vi "Handle EVENT.vi"(8 "error in (no error)":errorcluster, 9 "Message Loop Data (in)":T1, 10 "Cluster":T14 {"Message Codes" items=["HELLO"=1, "WELCOME"=2, "ABORT"=3, "GOODBYE"=6, "ERROR"=8, "PUBLISH"=16, "PUBLISHED"=17, "SUBSCRIBE"=32, "SUBSCRIBED"=33, "UNSUBSCRIBE"=34, "UNSUBSCRIBED"=35, "EVENT"=36, "CALL"=48, "RESULT"=59, "REGISTER"=64, "REGISTERED"=65, "UNREGISTER"=66, "UNREGISTERED"=67, "INVOCATION"=68, "YIELD"=70]}, 11 "reference":refnum<class "WAMP Client.lvclass">) -> (0 "error out":errorcluster, 1 "Message Loop Data (out)":T1, 3 "reference out":refnum<class "WAMP Client.lvclass">)   [LabVIEW 2020, in "wamplv.lvlib" / "WAMP Client.lvclass"]
uses:
  <vilib>/samangh/wamplv/WAMP Client/WAMP Client.lvclass
  <vilib>/samangh/wamplv/WAMP Client/TypeDef/WAMP Received Message.ctl
  <vilib>/samangh/wamplv/WAMP Message Codes.ctl
  <vilib>/samangh/wamplv/WAMP Client/TypeDef/Message Loop Shift Reg Data.ctl
  <vilib>/samangh/wamplv/WAMP Client/TypeDef/REGISTER Request Data.ctl
  <vilib>/samangh/wamplv/WAMP Client/TypeDef/REGISTERED or ERROR payload.ctl
  <vilib>/samangh/wamplv/WAMP Client/TypeDef/Combined error.ctl
  <vilib>/samangh/wamplv/WAMP Client/TypeDef/WAMP Error Payload.ctl
  <vilib>/samangh/wamplv/WAMP Client/TypeDef/INVOCATION payload.ctl
  <vilib>/samangh/wamplv/WAMP Client/TypeDef/Publish Requests Map.ctl
  <vilib>/samangh/wamplv/WAMP Client/TypeDef/PUBLISH Request Data.ctl
  <vilib>/samangh/wamplv/WAMP Client/TypeDef/PUBLISH Result.ctl
  <vilib>/samangh/wamplv/WAMP Client/TypeDef/Endpoint Data.ctl
  <vilib>/samangh/wamplv/WAMP Client/TypeDef/CALL Request Map.ctl
  <vilib>/samangh/wamplv/WAMP Client/TypeDef/CALL Request Data.ctl
  <vilib>/samangh/wamplv/WAMP Client/TypeDef/RESULT Payload.ctl
  <vilib>/samangh/wamplv/WAMP Client/TypeDef/SUBSCRIBE Requests Map.ctl
  <vilib>/samangh/wamplv/WAMP Client/TypeDef/SUBSCRIBE Request Data.ctl
  <vilib>/samangh/wamplv/WAMP Client/TypeDef/Subscribe Result.ctl
  <vilib>/samangh/wamplv/WAMP Client/TypeDef/Event Payload.ctl
  <vilib>/samangh/wamplv/WAMP Client/TypeDef/Subscriptions Map.ctl
  <vilib>/samangh/wamplv/WAMP Client/TypeDef/Subscription Details.ctl
  <vilib>/samangh/wamplv/WAMP Client/TypeDef/Unsubscribe Requests Map.ctl
  <vilib>/samangh/wamplv/WAMP Client/TypeDef/UNSUBSCRIBE Request Data.ctl
  <vilib>/samangh/wamplv/WAMP Client/TypeDef/UNSUBSCRIBE Result.ctl
  <vilib>/samangh/wamplv/WAMP Client/WAMP Client.lvclass/WAMP Client.ctl
  <vilib>/JDP Science/JSONtext/JSONtext.lvlib
panel:
  out "Details":string
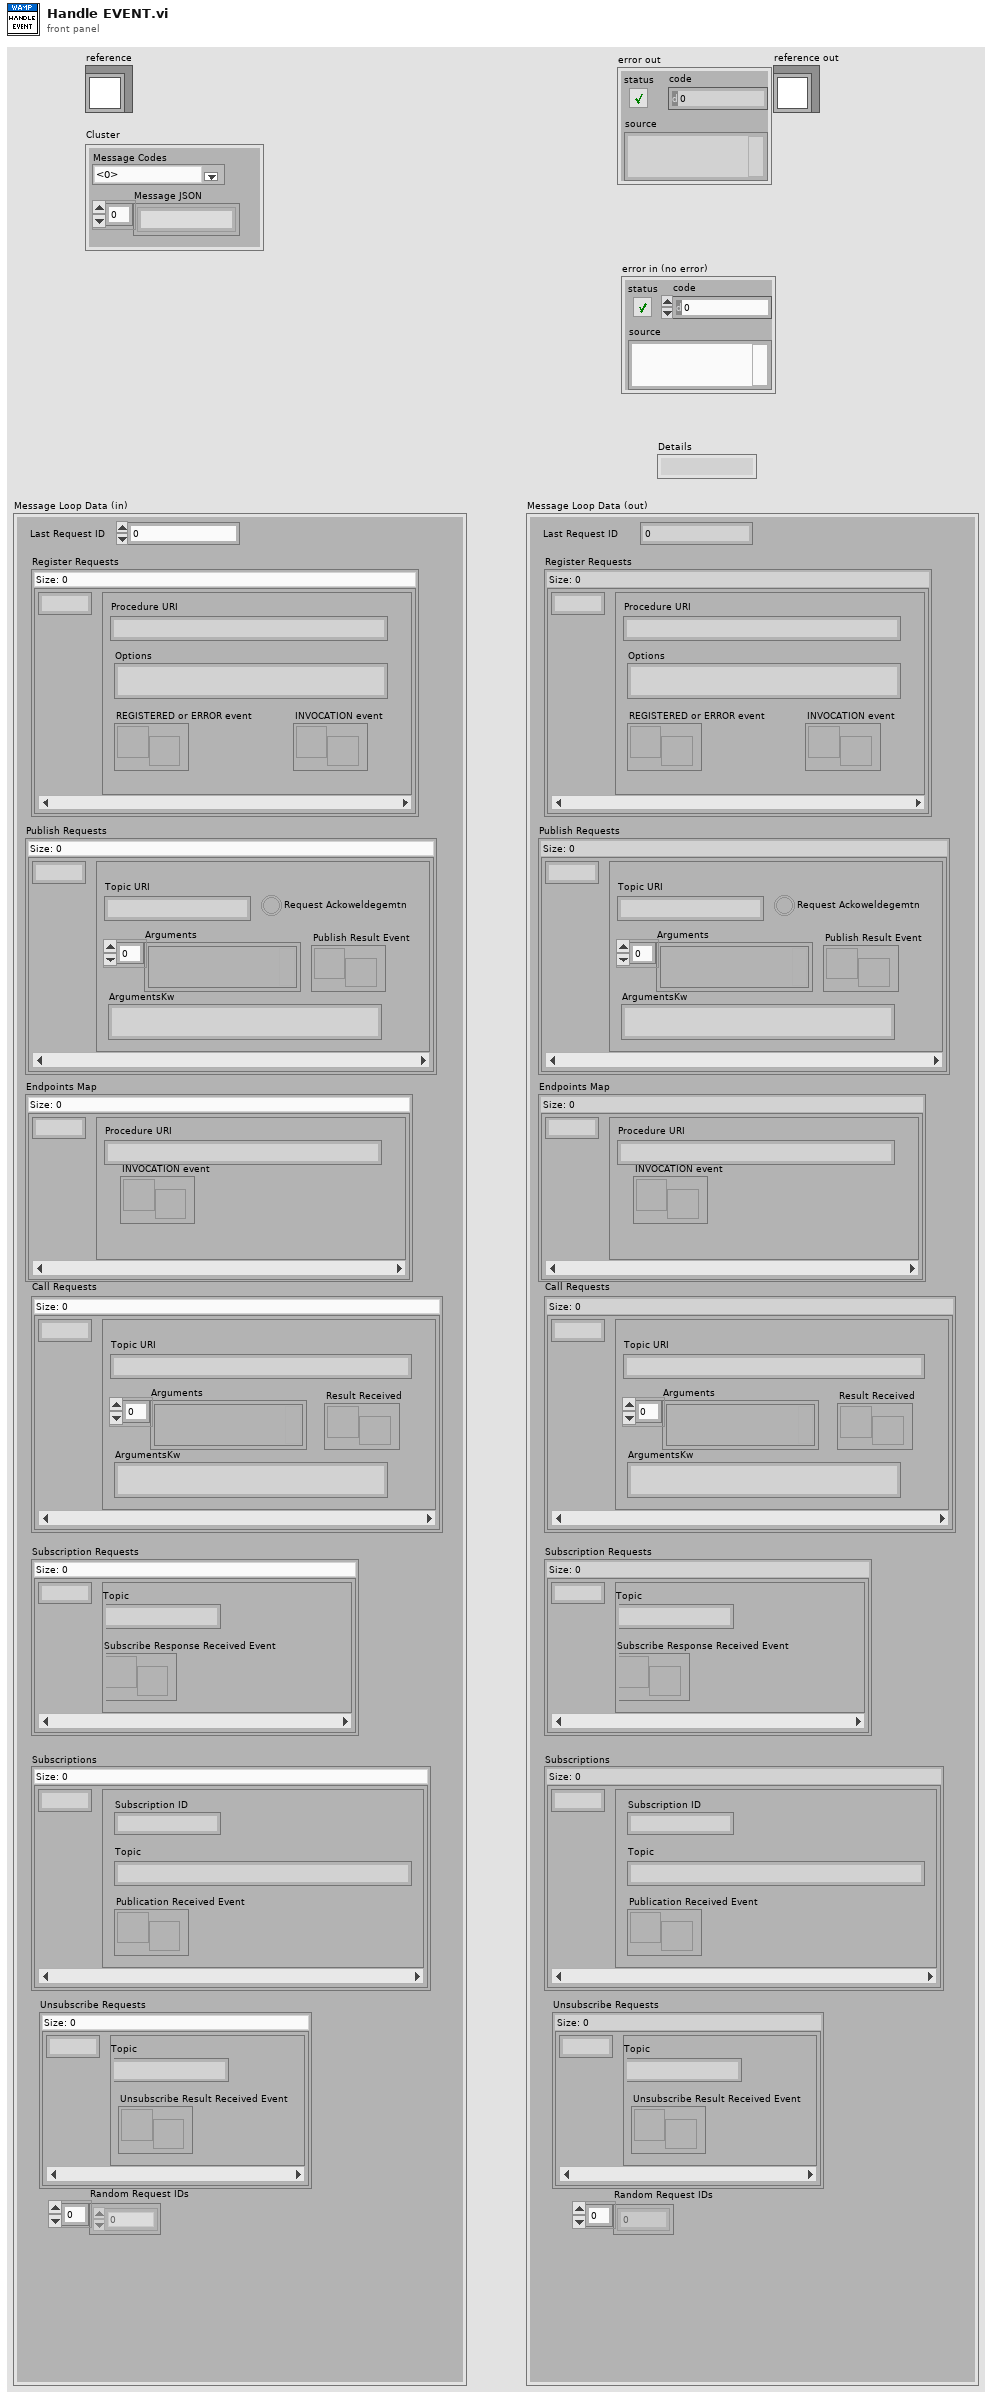
[diagram p1: front panel]
types:
  T1 = typedef "wamplv.lvlib/WAMP Client.lvclass/Message Loop Shift Reg Data.ctl" = cluster{"Last Request ID":u64, "Register Requests":map{u64, T2}, "Publish Requests":T3, "Endpoints Map":map{u64, T5}, "Call Requests":T6, "Subscription Requests":T8, "Subscriptions":T10, "Unsubscribe Requests":T12, "Random Request IDs":u64[]}
  T2 = typedef "wamplv.lvlib/WAMP Client.lvclass/REGISTER Request Data.ctl" = cluster{"Procedure URI":string, "Options":string, "REGISTERED or ERROR event":refnum<user-event>, "INVOCATION event":refnum<user-event>}
  T3 = typedef "wamplv.lvlib/WAMP Client.lvclass/Publish Requests Map.ctl" = map{u64, T4}
  T4 = typedef "wamplv.lvlib/WAMP Client.lvclass/PUBLISH Request Data.ctl" = cluster{"Topic URI":string, "Arguments":variant[], "ArgumentsKw":string, "Publish Result Event":refnum<user-event>, "Request Ackoweldegemtn":bool}
  T5 = typedef "wamplv.lvlib/WAMP Client.lvclass/Endpoint Data.ctl" = cluster{"Procedure URI":string, "INVOCATION event":refnum<user-event>}
  T6 = typedef "wamplv.lvlib/WAMP Client.lvclass/CALL Request Map.ctl" = map{u64, T7}
  T7 = typedef "wamplv.lvlib/WAMP Client.lvclass/CALL Request Data.ctl" = cluster{"Topic URI":string, "Arguments":variant[], "ArgumentsKw":string, "Result Received":refnum<user-event>}
  T8 = typedef "wamplv.lvlib/WAMP Client.lvclass/SUBSCRIBE Requests Map.ctl" = map{u64, T9}
  T9 = typedef "wamplv.lvlib/WAMP Client.lvclass/SUBSCRIBE Request Data.ctl" = cluster{"Topic":string, "Subscribe Response Received Event":refnum<user-event>}
  T10 = typedef "wamplv.lvlib/WAMP Client.lvclass/Subscriptions Map.ctl" = map{u64, T11}
  T11 = typedef "wamplv.lvlib/WAMP Client.lvclass/Subscription Details.ctl" = cluster{"Subscription ID":u64, "Topic":string, "Publication Received Event":refnum<user-event>}
  T12 = typedef "wamplv.lvlib/WAMP Client.lvclass/Unsubscribe Requests Map.ctl" = map{u64, T13}
  T13 = typedef "wamplv.lvlib/WAMP Client.lvclass/UNSUBSCRIBE Request Data.ctl" = cluster{"Topic":string, "Unsubscribe Result Received Event":refnum<user-event>}
  T14 = typedef "wamplv.lvlib/WAMP Client.lvclass/WAMP Received Message.ctl" = cluster{"Message JSON":string[], "Message Codes":T15}
  T15 = typedef "wamplv.lvlib/WAMP Client.lvclass/WAMP Message Codes.ctl" = u16
  T16 = typedef "wamplv.lvlib/WAMP Client.lvclass/Event Payload.ctl" = cluster{"Arguments Payload":string[], "ArgumentKw Payload":string, "Topic":string}
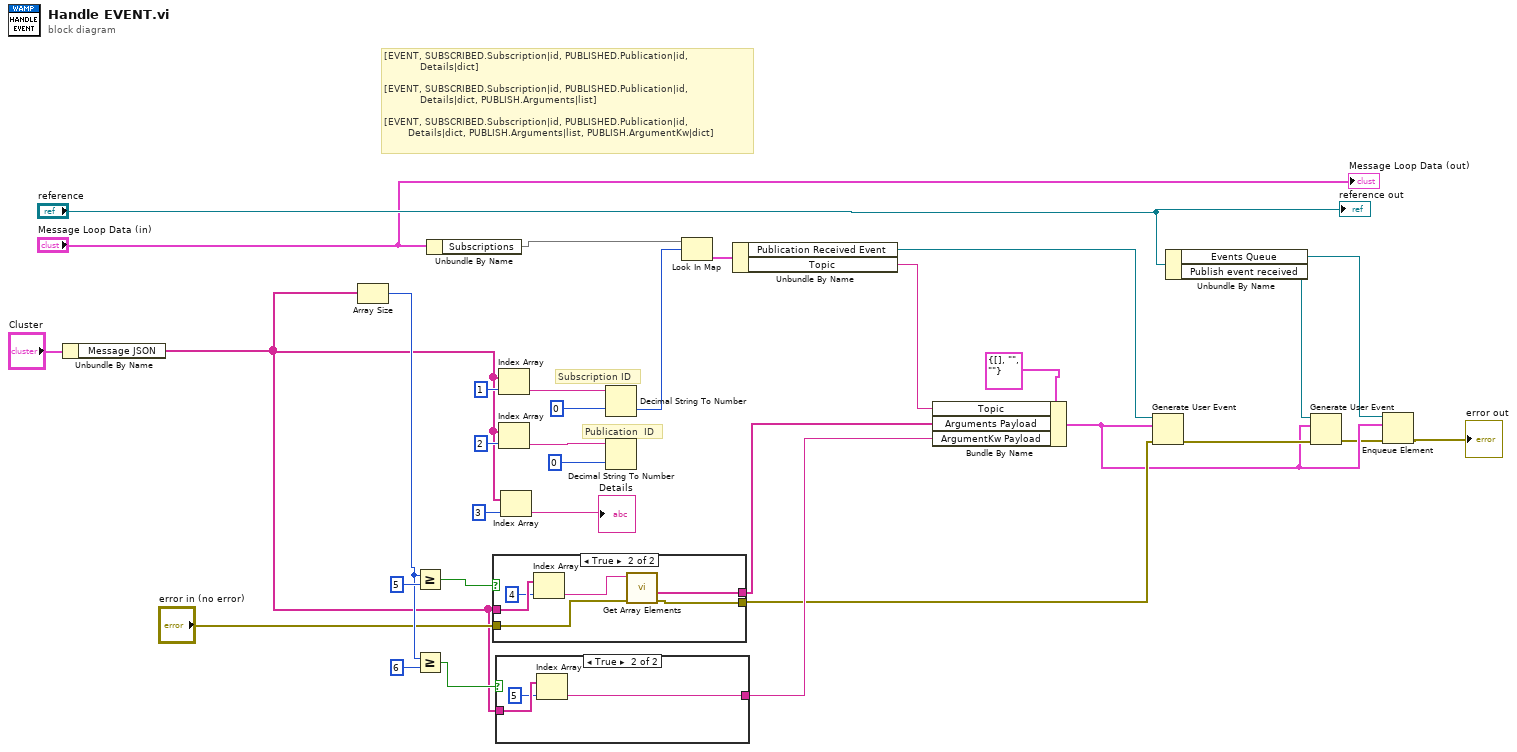
[diagram p0: block diagram]
diagram:
  # "[EVENT, SUBSCRIBED.Subscription|id, PUBLISHED.Publication|id,\n            Details|dict]\n\n[EVENT, SUBSCRIBED.Subscription|id, PUBLISHED.Publication|id,\n            Details|dict, PUBLISH.Arguments|list]\n\n[EVENT, SUBSCRIBED.Subscription|id, PUBLISHED.Publication|id,\n        Details|dict, PUBLISH.Arguments|list, PUBLISH.ArgumentKw|dict]"
  # "Publication  ID"
  # "Subscription ID"
  n1 = Unbundle By Name("Cluster") -> ("Message JSON"=w15:string[])
  n2 = Array Size(array=w15) -> (size(s)=w21:i32)
  n3 = Greater Or Equal?(x=w21, y=5) -> (x >= y?=w24:bool)
  n4 = Greater Or Equal?(x=w21, y=6) -> (x >= y?=w19:bool)
  n5 = Unbundle By Name("Message Loop Data (in)") -> ("Subscriptions"=w2:T10)
  n6 = case shown="True" w24 {
    tunnel: w15 -> [_ w39]
    tunnel: [_ w37] -> w23
    tunnel: "error in (no error)" -> [w34 w36]
    tunnel: [w34 w35] -> w17
    frame False {
    }
    frame True {
      n7 = Index Array(array=w39, index=4) -> (element=w40:string)
      n8 = call <vilib>:"Get Array Elements.vi"("error in (no error)"=w36, "JSON"=w40) -> ("error out"=w35:errorcluster, "<JSON>"=w37:string[])  [unwired: 7 in, 1 out]
    }
  }
  n9 = case shown="True" w19 {
    tunnel: w15 -> [_ w43]
    tunnel: [_ w41] -> w20
    frame False {
    }
    frame True {
      n10 = Index Array(array=w43, index=5) -> (element=w41:string)
    }
  }
  n11 = Index Array(array=w15, index=1) -> (element=w32:string)
  n12 = Index Array(array=w15, index=2) -> (element=w33:string)
  n13 = Index Array(array=w15, index=3) -> (element=→"Details":string)
  n14 = Decimal String To Number(string=w32, default (0L)=u64 0) -> (number=w14:u64)  [unwired: 1 in, 1 out]
  n15 = Decimal String To Number(string=w33, default (0L)=u64 0) -> ()  [unwired: 1 in, 2 out]
  n16 = Look In Map(map=w2, key=w14) -> (value=w13:T11)  [unwired: 1 in, 1 out]
  n17 = Unbundle By Name(w13) -> ("Publication Received Event"=w12:refnum<user-event>, "Topic"=w11:string)
  n18 = Bundle By Name(cluster=T16 {"Arguments Payload"=[], "ArgumentKw Payload"="", "Topic"=""} ("Cluster"), "Topic"=w11, "Arguments Payload"=w23, "ArgumentKw Payload"=w20) -> (w5:T16)
  n19 = Generate User Event(user event=w12, event data cluster=w5, error in=w17) -> (error out=w7:errorcluster)  [unwired: 1 in, 1 out]
  n20 = Unbundle By Name("reference") -> ("Events Queue"=w6:refnum<queue>, "Publish event received"=w9:refnum<user-event>)
  n21 = Generate User Event(user event=w9, event data cluster=w5, error in=w7) -> (error out=w4:errorcluster)  [unwired: 1 in, 1 out]
  n22 = Enqueue Element(queue=w6, element=w5, error in (no error)=w4) -> (error out=→"error out":errorcluster)  [unwired: 1 in, 2 out]
  "reference out" <- "reference"
  "Message Loop Data (out)" <- "Message Loop Data (in)"
